vi "FTW-SEQ-GetNextStep.vi"(8 "error in":errorcluster, 11 "Sequencer":refnum<class "FTW-Sequencer.lvclass">) -> (0 "error out":errorcluster, 1 "Job Data":string, 2 "Current Job":string, 3 "Sequencer out":refnum<class "FTW-Sequencer.lvclass">)   [LabVIEW 2015, in "FTW-Sequencer.lvclass"]
uses:
  FTW-Sequencer.lvclass
  FTW-Sequencer.lvclass/FTW-Sequencer.ctl
  Error/FTW-ERR-ThrowError.vi
panel:
  # "Inputs"
  # "Outputs"
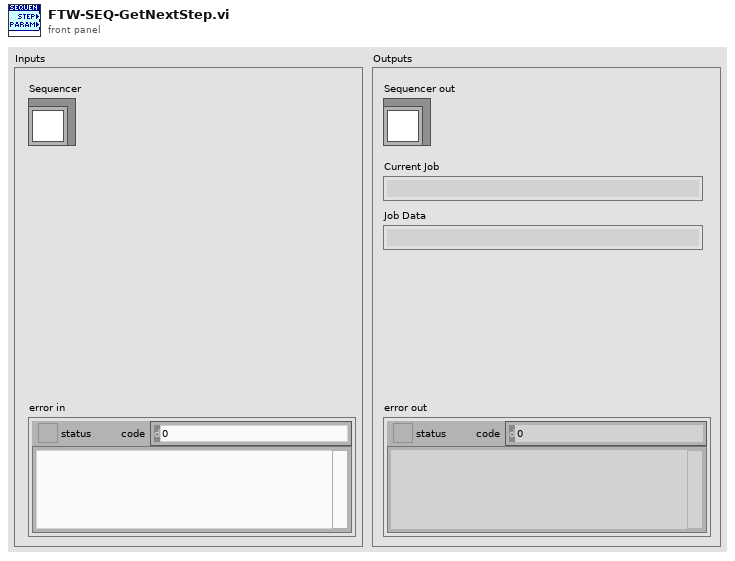
[diagram p1: front panel]
types:
  T1 = typedef "FTW-ERR-ExceptionType.ctl" = enum16{"No Error", "Error", "Warning"}
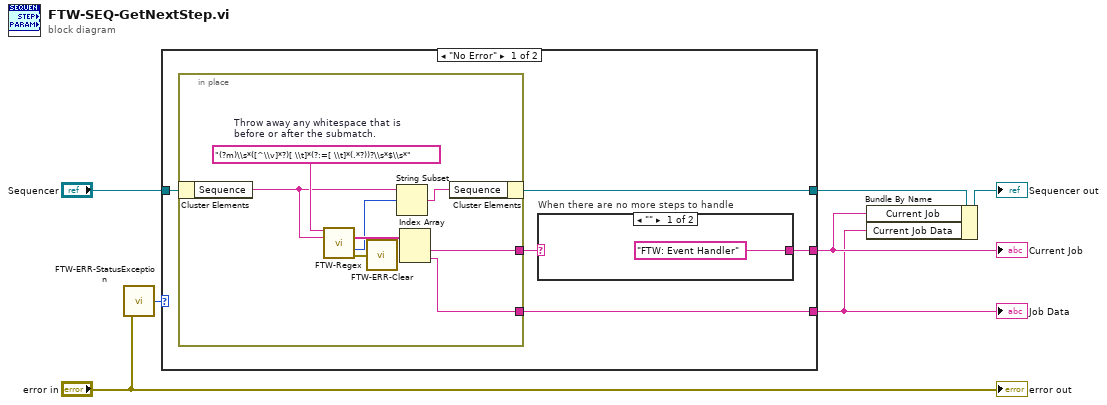
[diagram p0: block diagram]
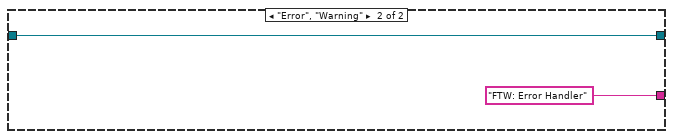
[diagram p3: hidden frame]
diagram:
  n1 = call "FTW-ERR-StatusException.vi"("error to check"="error in") -> ("Exception"=w5:T1)
  n2 = case shown="\"No Error\"" w5 {
    tunnel: "Sequencer" -> [w9 w24]
    tunnel: [w11 "FTW: Error Handler" ("submatch 1")] -> w2
    tunnel: [w8 w24] -> w6
    tunnel: [w10 _] -> w1
    frame "No Error" {
      n3 = in-place {
        in-place-border: [w18] -> w12
        in-place-border: [w17] -> w10
        w20 = "(?m)\\s*([^\\v]*?)[ \\t]*(?:=[ \\t]*(.*?))?\\s*$\\s*"  # Throw away any whitespace that is before or after the submatch.
        n4 = in-place-cluster #1(w9) -> ("Sequence"=w16:string)
        n5 = call "FTW-Regex.vi"("Regular Expression"=w20, "Input String"=w16) -> ("Submatches"=w19:string[], "Offset after Match"=w15:i32, "error out"=w13:errorcluster)  [unwired: 9 in, 2 out]
        n6 = call "FTW-ERR-Clear.vi"("error to snuff"=w13) -> ()  [unwired: 1 out]
        n7 = String Subset(string=w16, offset (0)=w15) -> (substring=w14:string)  [unwired: 1 in]
        n8 = Index Array(array=w19) -> (element #1=w18:string, element #2=w17:string)  [unwired: 2 in]
        n9 = in-place-cluster #1("Sequence"=w14) -> (w8:refnum<class "FTW-Sequencer.lvclass">)
      }
      n10 = case "When there are no more steps to handle" shown="\"\"" w12 {
        selector: w12 -> [_ w22]
        tunnel: ["FTW: Event Handler" w22] -> w11
        frame "" {
        }
        frame Default {
        }
      }
    }
    frame "Error", "Warning" {
    }
  }
  "Current Job" <- w2
  "Job Data" <- w1
  n11 = Bundle By Name(cluster=w6, "Current Job"=w2, "Current Job Data"=w1) -> (→"Sequencer out":refnum<class "FTW-Sequencer.lvclass">)
  "error out" <- "error in"
